vi "SetComboBoxFlatStyle.vi"(0 "reference in":refnum<class "DataGridView.lvclass">, 5 "FlatStyle":i32(ring) items=["Flat", "Popup", "Standard", "System"], 11 "error in (no error)":errorcluster) -> (4 "reference out":refnum<class "DataGridView.lvclass">, 15 "error out":errorcluster)   [LabVIEW 2018, in "DataGridView.lvclass"]
uses:
  DataGridView.lvclass
  System.Windows.Forms
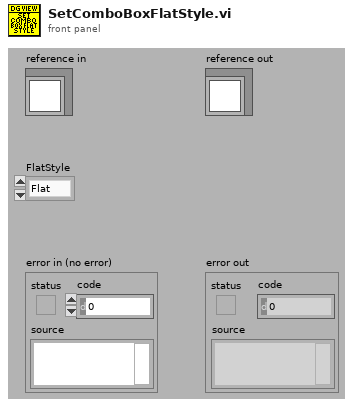
[diagram p1: front panel]
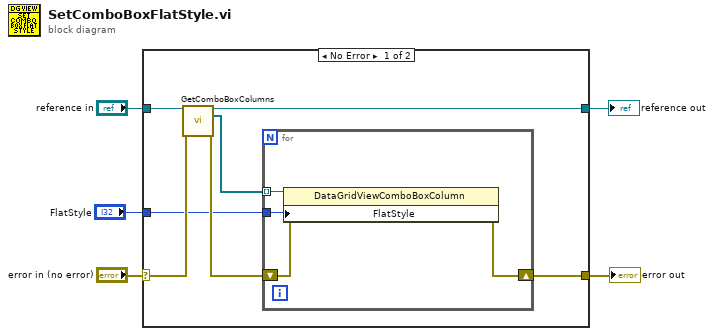
[diagram p0: block diagram]
diagram:
  n1 = case shown="No Error" "error in (no error)" {
    selector: "error in (no error)" -> [w12 w18]
    tunnel: [w8 w18] -> w4
    tunnel: [w10 w17] -> w2
    tunnel: "reference in" -> [w11 w17]
    tunnel: "FlatStyle" -> [w6 _]
    frame No Error {
      n2 = call "GetComboBoxColumns.vi"("reference in"=w11, "error in (no error)"=w12) -> ("reference out"=w10:refnum<class "DataGridView.lvclass">, "ComboBoxColumns"=w7:refnum<k24>[], "error out"=w9:errorcluster)  [unwired: 11 in]
      n3 = for {
        shift-right: [w15] -> w8
        shift-left: w9 -> [w16]
        tunnel: w7 -> [w14] mode=indexing
        tunnel: w6 -> [w13]
        n4 = property class="DataGridViewComboBoxColumn"(reference=w14, error in=w16, "FlatStyle"=w13) -> (error out=w15:errorcluster)  [unwired: 1 out]
      }
    }
    frame Error {
    }
  }
  "error out" <- w4
  "reference out" <- w2
